vi "estimate current pos and vel kalman.vi"(9 "feedback lowpass f":dbl=30.0 format="%0.4f", 11 "kalman updates":T1[](array[typedef])) -> (4 "current velocity":dbl[](array[numeric]), 5 "current position":dbl[](array[numeric]))   [LabVIEW 2010]
uses:
  kalman_result_scaled.ctl
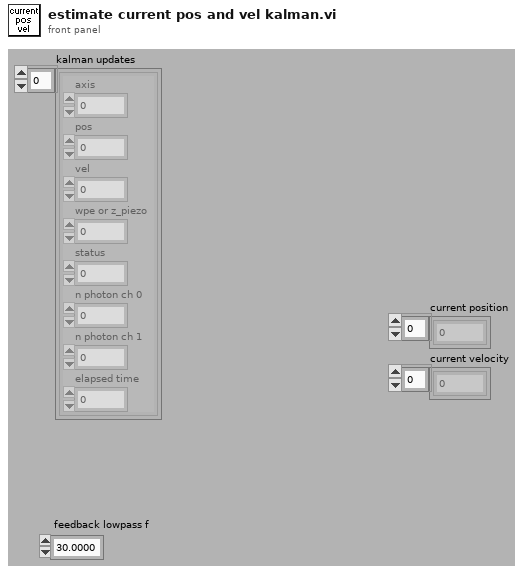
[diagram p1: front panel]
types:
  T1 = typedef "kalman_result_scaled.ctl" = cluster{"axis":u8, "pos":dbl, "vel":dbl, "wpe or z_piezo":dbl, "status":u32, "n photon ch 0":u32, "n photon ch 1":u32, "elapsed time":dbl}
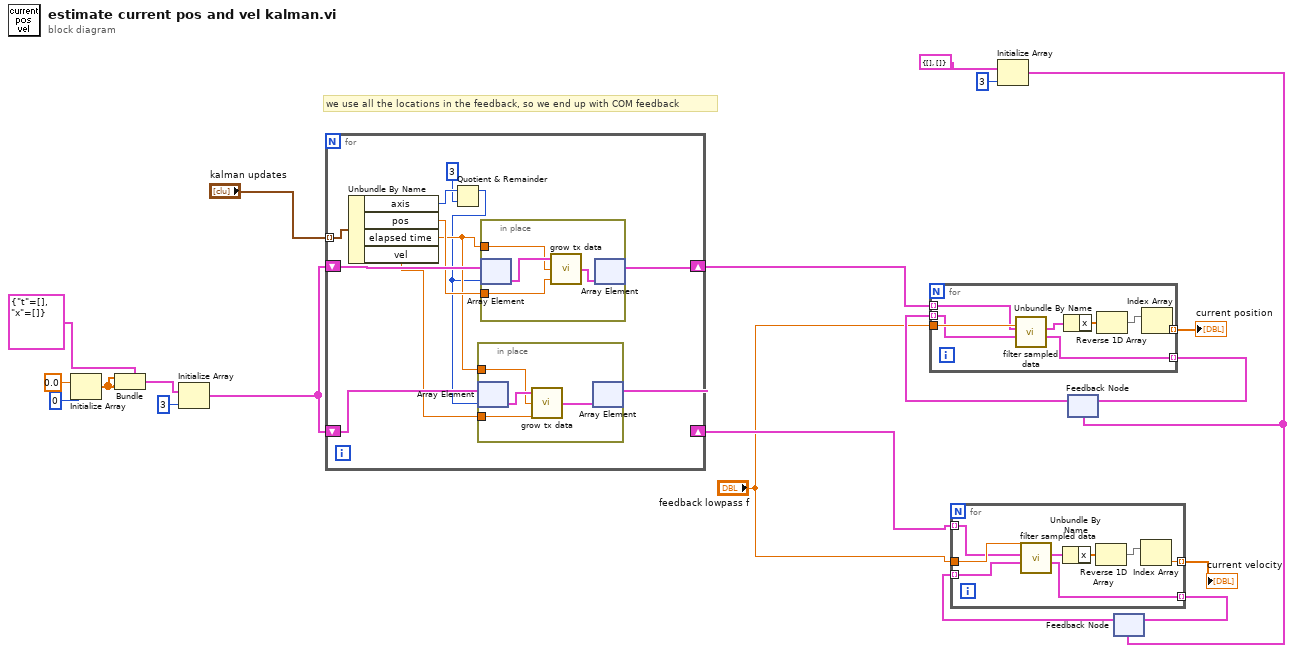
[diagram p0: block diagram]
diagram:
  # "we use all the locations in the feedback, so we end up with COM feedback"
  n1 = Initialize Array(0.0 ("element"), 0 ("dimension size")) -> (w13:dbl[])
  n2 = Bundle(cluster=cluster{"t":dbl[], "x":dbl[]} {"t"=[], "x"=[]} ("xt val"), "t"=w13, "x"=w13) -> (w6:cluster{"t":dbl[], "x":dbl[]})
  n3 = Initialize Array(w6, 3 ("dimension size")) -> (w19:cluster{"t":dbl[], "x":dbl[]}[])
  n4 = for {
    tunnel: "kalman updates" -> [w24] mode=indexing
    shift-right: [w29] -> w5
    shift-left: w19 -> [w31]
    shift-right: [w25] -> w18
    shift-left: w19 -> [w28]
    n5 = Unbundle By Name(w24) -> ("axis"=w23:u8, "pos"=w30:dbl, "elapsed time"=w27:dbl, "vel"=w26:dbl)
    n6 = Quotient & Remainder(x=w23, y=u8 3) -> (x-y*floor(x/y)=w21:u8)  [unwired: 1 out]
    n7 = in-place {
      in-place-border: w27 -> [w34]
      in-place-border: w26 -> [w33]
      n8 = in-place-array #1(w28, w21) -> (w35:cluster{"t":dbl[], "x":dbl[]})
      n9 = call "grow tx data.vi"("value"=w33, "time"=w34, "tx data in"=w35) -> ("tx data out"=w32:cluster{"t":dbl[], "x":dbl[]})
      n10 = in-place-array #1(w32) -> (w25:cluster{"t":dbl[], "x":dbl[]}[])  [unwired: 1 out]
    }
    n11 = in-place {
      in-place-border: w27 -> [w38]
      in-place-border: w30 -> [w37]
      n12 = in-place-array #2(w31, w21) -> (w39:cluster{"t":dbl[], "x":dbl[]})
      n13 = call "grow tx data.vi"("value"=w37, "time"=w38, "tx data in"=w39) -> ("tx data out"=w36:cluster{"t":dbl[], "x":dbl[]})
      n14 = in-place-array #2(w36) -> (w29:cluster{"t":dbl[], "x":dbl[]}[])  [unwired: 1 out]
    }
  }
  n15 = Initialize Array(cluster{"t":dbl[], "x":dbl[]} {"t"=[], "x"=[]} ("xt val"), 3 ("dimension size")) -> (w7:cluster{"t":dbl[], "x":dbl[]}[])
  n16 = feedback #3(w7) -> (w10:cluster{"t":dbl[], "x":dbl[]}[])
  n17 = for {
    tunnel: w5 -> [w46] mode=indexing
    tunnel: [w40] -> w11 mode=indexing
    tunnel: w10 -> [w45] mode=indexing
    tunnel: "feedback lowpass f" -> [w47]
    tunnel: [w41] -> w4 mode=indexing
    n18 = call "filter sampled data.vi"("low cutoff freq: fl"=w47, "last data set"=w45, "t x data"=w46) -> ("current data set"=w40:cluster{"t":dbl[], "x":dbl[]}, "t x data filetered"=w44:cluster{"t":dbl[], "x":dbl[]})  [unwired: 7 in]
    n19 = Unbundle By Name(w44) -> ("x"=w42:dbl[])
    n20 = Reverse 1D Array(array=w42) -> (reversed array=w43:dbl[])
    n21 = Index Array(array=w43) -> (element=w41:dbl)  [unwired: 1 in]
  }
  "current position" <- w4
  n22 = feedback-in #3(w11) -> ()
  n23 = feedback #4(w7) -> (w8:cluster{"t":dbl[], "x":dbl[]}[])
  n24 = for {
    tunnel: w18 -> [w54] mode=indexing
    tunnel: [w48] -> w9 mode=indexing
    tunnel: w8 -> [w53] mode=indexing
    tunnel: "feedback lowpass f" -> [w55]
    tunnel: [w49] -> w2 mode=indexing
    n25 = call "filter sampled data.vi"("low cutoff freq: fl"=w55, "last data set"=w53, "t x data"=w54) -> ("current data set"=w48:cluster{"t":dbl[], "x":dbl[]}, "t x data filetered"=w50:cluster{"t":dbl[], "x":dbl[]})  [unwired: 7 in]
    n26 = Unbundle By Name(w50) -> ("x"=w51:dbl[])
    n27 = Reverse 1D Array(array=w51) -> (reversed array=w52:dbl[])
    n28 = Index Array(array=w52) -> (element=w49:dbl)  [unwired: 1 in]
  }
  "current velocity" <- w2
  n29 = feedback-in #4(w9) -> ()
